vi "first_project.vi"() -> ()   [LabVIEW 2018]
panel:
  in  "VISA resource name":refnum<visa-resource-name>="ASRL34::INSTR"
  in  "is PWM?":bool
  in  "Capture Range":u32=1 min=1 max=5 step=1
  in  "Capture Mode":u32(ring) items=["Auto Capture", "Manual Capture", "PWM Capture"]
  in  "Capture":bool
  in  "QUIT":bool
  out "Led Analyser Data":string[][](table)
  in  "XY":bool
  in  "RGB-Int":bool
  in  "Hue-Sat":bool
  # "NOTE: remember plug-in the Led Analyser\nbefore run this VI and to change the\nVISA resource name in the panel"
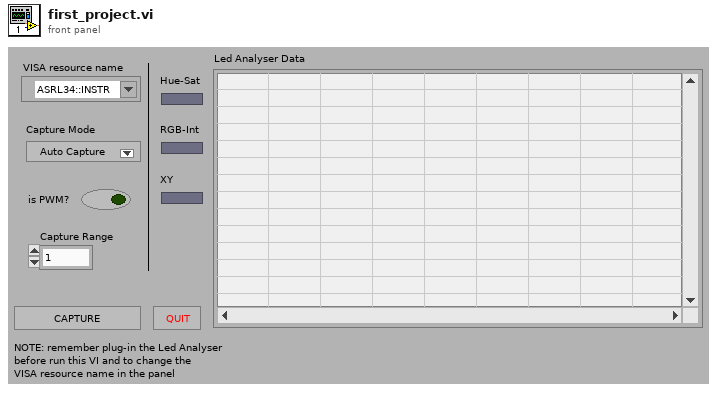
[diagram p1: front panel]
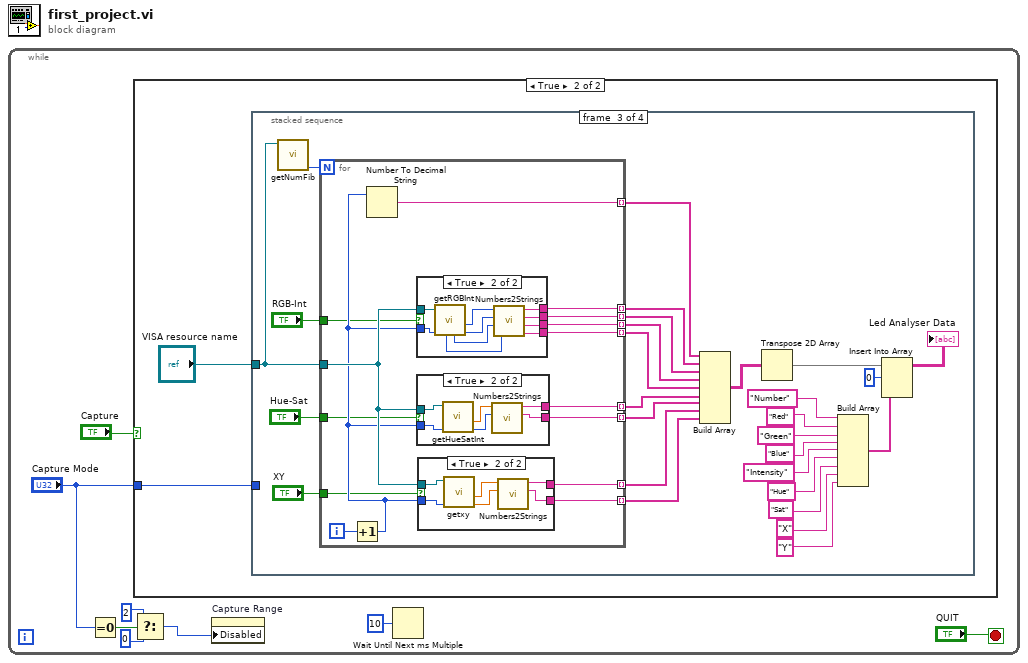
[diagram p0: block diagram]
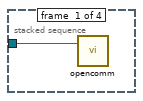
[diagram p3: hidden frame]
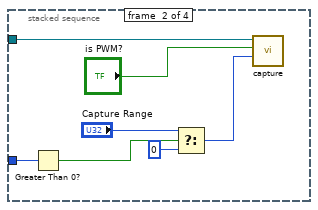
[diagram p4: hidden frame]
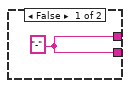
[diagram p5: hidden frame]
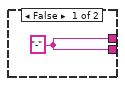
[diagram p6: hidden frame]
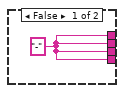
[diagram p7: hidden frame]
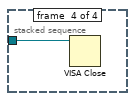
[diagram p8: hidden frame]
diagram:
  n1 = while {
    stop <- "QUIT" stop-if-true
    n2 = Equal To 0?(x="Capture Mode") -> (x = 0?=w5:bool)
    n3 = case shown="True" "Capture" {
      tunnel: "Capture Mode" -> [_ w9]
      frame False {
      }
      frame True {
        n4 = stacked-sequence {
          tunnel: "VISA resource name" -> [w11 w18 w19 w87]
          tunnel: w9 -> [_ w16 _ _]
          frame #0 {
            n5 = call "opencomm.vi"("VISA resource name"=w11) -> ()  [unwired: 3 in, 2 out]
          }
          frame #1 {
            n6 = Greater Than 0?(x=w16) -> (x > 0?=w13:bool)
            n7 = Select(t="Capture Range", s=w13, f=u32 0) -> (s? t:f=w15:u32)
            n8 = call "capture.vi"("Capture Range (0, auto)"=w15, "isPWM (no)"="is PWM?", "VISA resource name"=w18) -> ()  [unwired: 3 in, 2 out]
          }
          frame #2 {
            n9 = call "getNumFib.vi"("VISA resource name"=w19) -> ("Fiber Count"=w20:i32)  [unwired: 4 in, 2 out]
            n10 = for {
              N: w20 -> [_]
              tunnel: w19 -> [w61]
              tunnel: [w58] -> w42 mode=indexing
              tunnel: [w57] -> w43 mode=indexing
              tunnel: [w56] -> w44 mode=indexing
              tunnel: [w55] -> w45 mode=indexing
              tunnel: [w54] -> w46 mode=indexing
              tunnel: [w53] -> w40 mode=indexing
              tunnel: [w52] -> w39 mode=indexing
              tunnel: [w51] -> w38 mode=indexing
              tunnel: [w50] -> w37 mode=indexing
              tunnel: "RGB-Int" -> [w49]
              tunnel: "Hue-Sat" -> [w48]
              tunnel: "XY" -> [w47]
              i -> [w60]
              n11 = Increment(x=w60) -> (x+1=w59:i32)
              n12 = Number To Decimal String(number=w59) -> (decimal integer string=w58:string)  [unwired: 1 in]
              n13 = case shown="True" w49 {
                tunnel: w61 -> [_ w86]
                tunnel: w59 -> [_ w85]
                tunnel: [w76 w84] -> w57
                tunnel: [w76 w83] -> w56
                tunnel: [w76 w82] -> w55
                tunnel: [w76 w81] -> w54
                frame False {
                  w76 = "-"
                }
                frame True {
                  n14 = call "getRGBInt.vi"("Fiber Num"=w85, "VISA resource name"=w86) -> ("Green"=w79:u8, "Red"=w80:u8, "Blue"=w78:u8, "Intensity"=w77:u32)  [unwired: 4 in, 2 out]
                  n15 = call "Numbers2Strings.vi"("Number 4"=w77, "Number 3"=w78, "Number 2"=w79, "Number"=w80) -> ("Numeric String 4"=w81:string, "Numeric String 3"=w82:string, "Numeric String 2"=w83:string, "Numeric String 1"=w84:string)
                }
              }
              n16 = case shown="True" w48 {
                tunnel: w61 -> [_ w75]
                tunnel: w59 -> [_ w74]
                tunnel: [w69 w73] -> w53
                tunnel: [w69 w72] -> w52
                frame False {
                  w69 = "-"
                }
                frame True {
                  n17 = call "getHueSatInt.vi"("Fiber Num"=w74, "VISA resource name"=w75) -> ("Saturation"=w70:u32, "Hue"=w71:dbl)  [unwired: 3 in, 3 out]
                  n18 = call "Numbers2Strings.vi"("Number 2"=w70, "Number"=w71) -> ("Numeric String 2"=w72:string, "Numeric String 1"=w73:string)  [unwired: 2 in, 2 out]
                }
              }
              n19 = case shown="True" w47 {
                tunnel: w61 -> [_ w68]
                tunnel: w59 -> [_ w67]
                tunnel: [w62 w66] -> w51
                tunnel: [w62 w65] -> w50
                frame False {
                  w62 = "-"
                }
                frame True {
                  n20 = call "getxy.vi"("Fiber Num"=w67, "VISA resource name"=w68) -> ("y (CIE1931)"=w63:dbl, "x (CIE1931)"=w64:dbl)  [unwired: 2 in, 2 out]
                  n21 = call "Numbers2Strings.vi"("Number 2"=w63, "Number"=w64) -> ("Numeric String 2"=w65:string, "Numeric String 1"=w66:string)  [unwired: 2 in, 2 out]
                }
              }
            }
            n22 = Build Array(w42, w43, w44, w45, w46, w40, w39, w38, w37) -> (w41:string[][])
            n23 = Transpose 2D Array(2D array=w41) -> (transposed array=w26:string[][])
            n24 = Build Array("Number", "Red", "Green", "Blue", "Intensity", "Hue", "Sat", "X", "Y") -> (w25:string[])
            n25 = Insert Into Array(array=w26, index (row)=0 ("Index (row)"), new element=w25) -> (→"Led Analyser Data":string[][])  [unwired: 1 in]
          }
          frame #3 {
            n26 = VISA Close(VISA resource name=w87) -> ()  [unwired: 1 in, 1 out]
          }
        }
      }
    }
    n27 = Select(t=u16 2 ("f"), s=w5, f=u16 0) -> (s? t:f=w1:u16)
    n28 = property on="Capture Range" class="DigNum (strict)"("Disabled"=w1) -> ()  [unwired: 2 in, 2 out]
    n29 = Wait Until Next ms Multiple(millisecond multiple=u32 10) -> ()  [unwired: 1 out]
  }
